vi "Elf2DataRecord.vi"(11 "Elf file":path) -> (3 "DataRecord":T1 {"Address" format="%.0x"; "Data" format="%.0x"})   [LabVIEW 2016]
uses:
  DataControl.ctl
panel:
  out "element":cluster{"Address":u32, "Data":u32} {"Address" format="%.0x"}
  out "size(s)":i32
  out "filename without extension":string
  out "resulting string":string
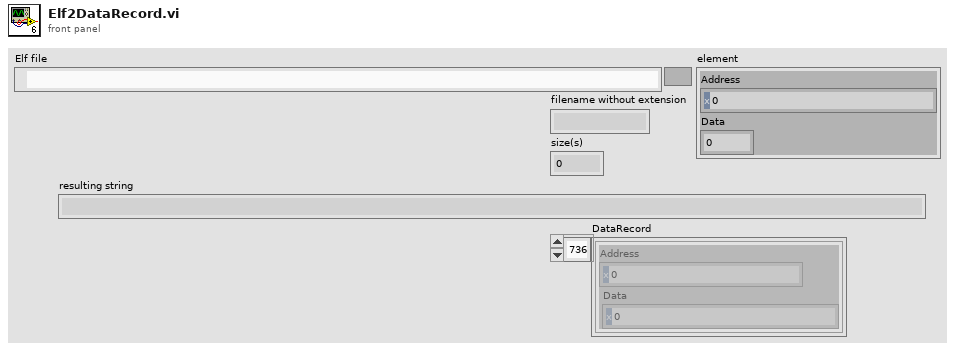
[diagram p1: front panel]
types:
  T1 = typedef "DataControl.ctl" = cluster{"Address":u32, "Data":u32}[]
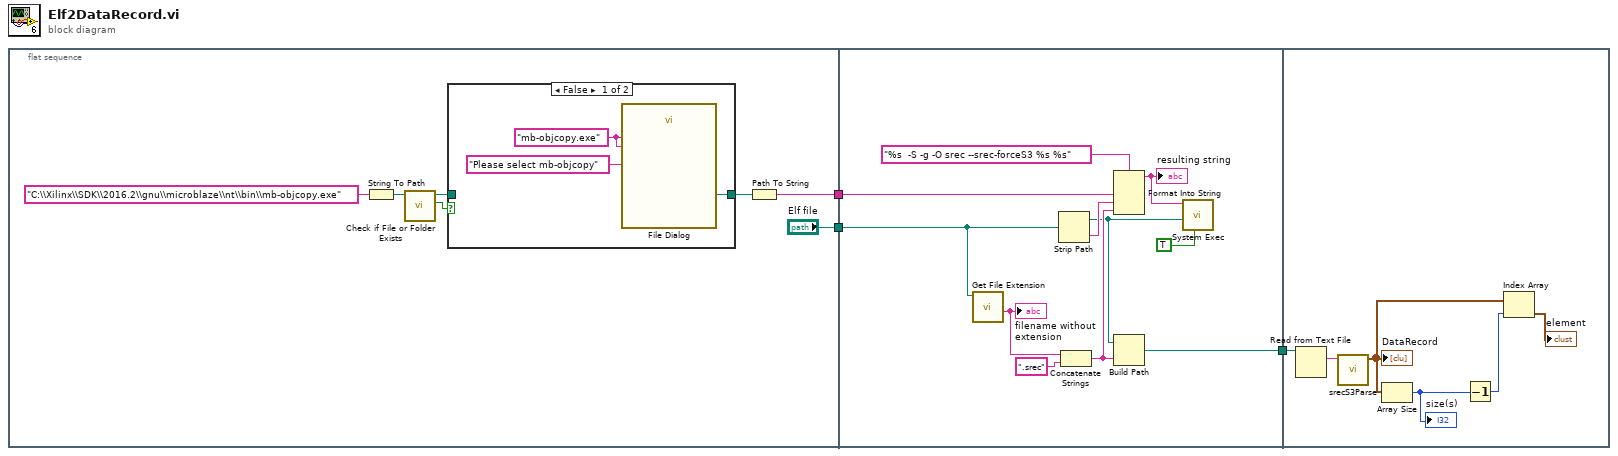
[diagram p0: block diagram]
diagram:
  n1 = flat-sequence {
    tunnel: ["Elf file"] -> w3
    tunnel: [w4] -> w2
    tunnel: w3 -> [w22]
    tunnel: w2 -> [w23]
    tunnel: [w15] -> w1
    tunnel: w1 -> [w31]
    frame #0 {
      n2 = String To Path(string="C:\\Xilinx\\SDK\\2016.2\\gnu\\microblaze\\nt\\bin\\mb-objcopy.exe") -> (path=w9:path)
      n3 = call <vilib>:"Check if File or Folder Exists.vi"("path"=w9) -> ("file or folder exists?"=w8:bool, "dup path"=w7:path)  [unwired: 8 in, 1 out]
      n4 = case shown="False" w8 {
        tunnel: w7 -> [_ w14]
        tunnel: [w13 w14] -> w5
        frame False {
          w11 = "mb-objcopy.exe" ("pattern label")
          n5 = call "File Dialog"("prompt"="Please select mb-objcopy", "pattern (all files)"=w11, "pattern label"=w11) -> ("selected path"=w13:path)  [unwired: 9 in, 3 out]
        }
        frame True {
        }
      }
      n6 = Path To String(path=w5) -> (string=w4:string)
    }
    frame #1 {
      n7 = call <vilib>:"Get File Extension.vi"("file"=w22) -> ("filename without extension"=w21:string)  [unwired: 6 in, 4 out]
      "filename without extension" <- w21
      n8 = Strip Path(path=w22) -> (stripped path=w16:path, name=w24:string)
      n9 = Concatenate Strings(w21, ".srec" ("string")) -> (w17:string)
      n10 = Format Into String(format string="%s  -S -g -O srec --srec-forceS3 %s %s", w23, w24, w17) -> (resulting string=w18:string)  [unwired: 2 in, 1 out]
      "resulting string" <- w18
      n11 = Build Path(base path=w16, name or relative path=w17) -> (appended path=w15:path)
      n12 = call <vilib>:"System Exec.vi"("run minimized? (F)"=TRUE, "working directory"=w16, "command line"=w18) -> ()  [unwired: 5 in, 4 out]
    }
    frame #2 {
      n13 = Read from Text File(file (use dialog)=w31) -> (text=w30:string)  [unwired: 3 in, 3 out]
      n14 = call "srecS3Parse.vi"("SrecS3"=w30) -> ("DataRecord"=w29:cluster{"Address":u32, "Data":u32}[])  [unwired: 10 in]
      "DataRecord" <- w29
      n15 = Array Size(array=w29) -> (size(s)=w28:i32)
      "size(s)" <- w28
      n16 = Decrement(x=w28) -> (x-1=w27:i32)
      n17 = Index Array(array=w29, index=w27) -> (element=→"element":cluster{"Address":u32, "Data":u32})
    }
  }
